vi "SendBackChannelMetadataTrigger.vi"(8 "error in":errorcluster, 11 "rdma session in":refnum<k21>) -> (0 "error out":errorcluster, 3 "rdma session out":refnum<k21>)   [LabVIEW 2021]
uses:
  2c4f7a5f-5cb5-431a-8e2b-0a6c60a0d62e.vi
  2c4f7a5f-5cb5-431a-8e2b-0a6c60a0d62e.vi/c7caca0c-161a-4e5d-b028-879c1e2dca2f.vi
  2c4f7a5f-5cb5-431a-8e2b-0a6c60a0d62e.vi/72e164ce-c078-45d0-ba5f-a1d3dac130e9.vi
  <vilib>/rdma/rdma.llb/RDMA Acquire Send Buffer U8.vi
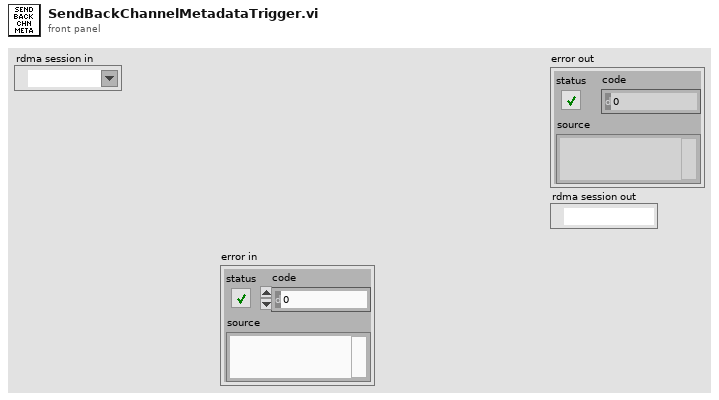
[diagram p1: front panel]
types:
  T1 = cluster{"requestType":u32, "backChannelMajorVersion":u16, "backChannelMinorVersion":u16, "debugInfoServerEnabled":u8, "debugInfoServerAddressSize":u32, "debugInfoServerPort":u16}
  T2 = enum16{"big-endian, network order", "native, host order", "little-endian"}
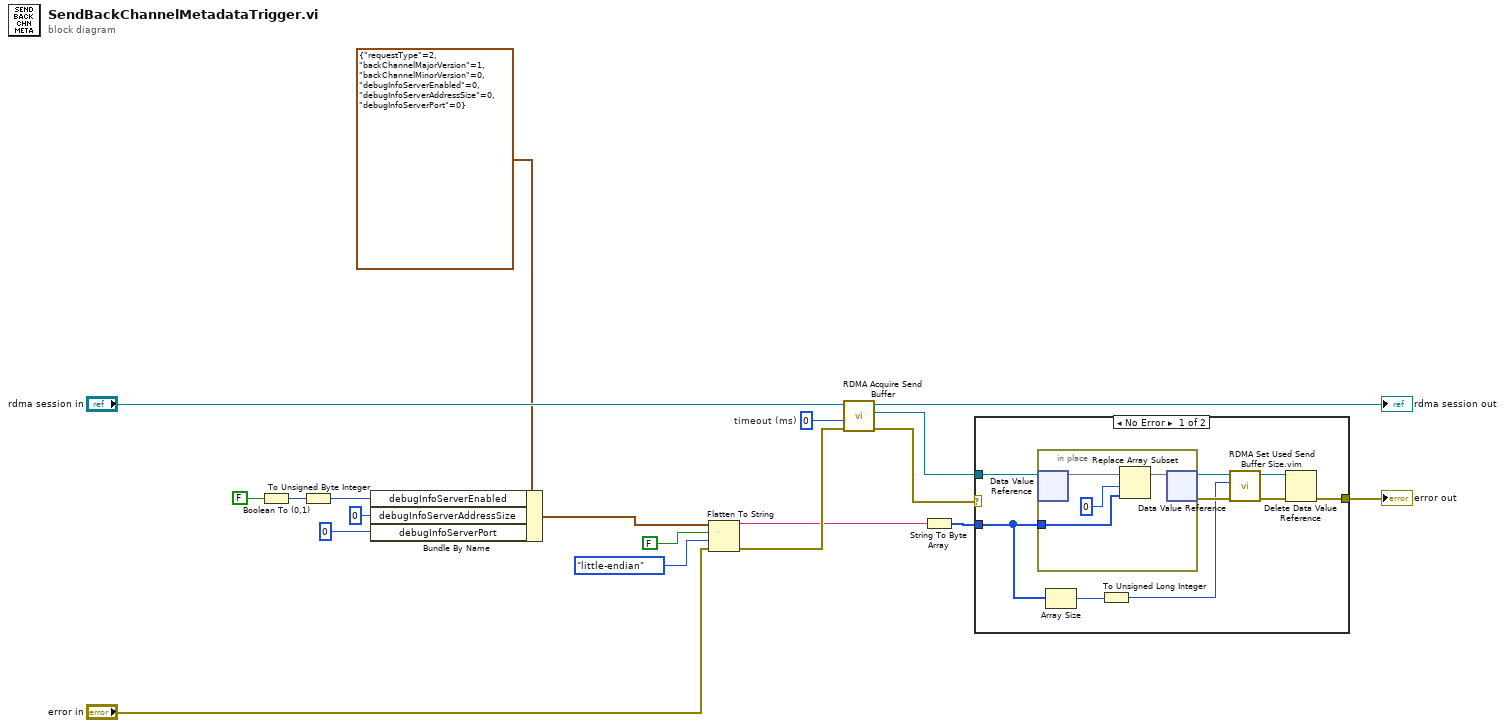
[diagram p0: block diagram]
diagram:
  w18 = 0  # timeout (ms)
  n1 = Boolean To (0,1)(Boolean=FALSE) -> (0, 1=w7:i16)
  n2 = To Unsigned Byte Integer(number=w7) -> (unsigned 8bit integer=w6:u8)
  n3 = Bundle By Name(cluster=T1 {"requestType"=2, "backChannelMajorVersion"=1, "backChannelMinorVersion"=0, "debugInfoServerEnabled"=0, "debugInfoServerAddressSize"=0, "debugInfoServerPort"=0}, "debugInfoServerEnabled"=w6, "debugInfoServerAddressSize"=u32 0, "debugInfoServerPort"=u16 0) -> (w14:T1)
  n4 = Flatten To String(anything=w14, prepend array or string size? (T)=FALSE, byte order (0:big-endian, network order)=T2."little-endian", error in (no error)="error in") -> (data string=w2:string, error out=w9:errorcluster)  [unwired: 1 out]
  n5 = call-poly <vilib>:"RDMA Acquire Send Buffer.vi"("error in"=w9, "timeout (ms)"=w18, "rdma session in"="rdma session in") -> ("error out"=w17:errorcluster, "edvr"=w15:refnum<data-value>, "rdma session out"=→"rdma session out":refnum<k21>)  [unwired: 6 in]
  n6 = String To Byte Array(string=w2) -> (unsigned byte array=w11:u8[])
  n7 = case shown="No Error" w17 {
    selector: w17 -> [_ w33]
    tunnel: w15 -> [w28 _]
    tunnel: w11 -> [w23 _]
    tunnel: [w20 w33] -> w10
    frame No Error {
      n8 = in-place {
        in-place-border: w23 -> [w31]
        n9 = in-place-dvr #1(w28) -> (w32:u8[])  [unwired: 1 out]
        n10 = Replace Array Subset(array=w32, new element=w31, index=0) -> (w29:u8[])
        n11 = in-place-dvr #1(w29) -> (w27:refnum<data-value>, w25:errorcluster)
      }
      n12 = Array Size(array=w23) -> (size(s)=w22:i32)
      n13 = To Unsigned Long Integer(number=w22) -> (unsigned 32bit integer=w21:u32)
      n14 = call "RDMA Set Used Send Buffer Size.vim"("error in"=w25, "used send buffer size"=w21, "edvr in"=w27) -> ("error out"=w24:errorcluster, "edvr out"=w26:refnum<data-value>)  [unwired: 7 in]
      n15 = Delete Data Value Reference(data value reference=w26, error in=w24) -> (error out=w20:errorcluster)  [unwired: 1 out]
    }
    frame Error {
    }
  }
  "error out" <- w10
